vi "Write actor.vi"(8 "error in (no error)":errorcluster, 10 "actor":refnum<class "Actor.lvclass">, 11 "[MV] Key Certify in":refnum<class "[MV] Key Certify.lvclass">) -> (0 "error out":errorcluster, 3 "[MV] Key Certify out":refnum<class "[MV] Key Certify.lvclass">)   [LabVIEW 2023, in "[MV] Key Certify.lvlib" / "[MV] Key Certify.lvclass"]
uses:
  [MV] Key Certify.lvclass
  [MV] Key Certify.lvclass/[MV] Key Certify.ctl
  <vilib>/ActorFramework/Actor/Actor.lvclass
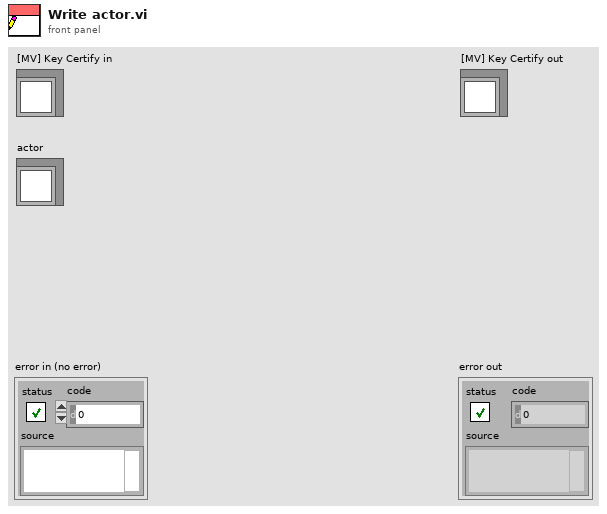
[diagram p1: front panel]
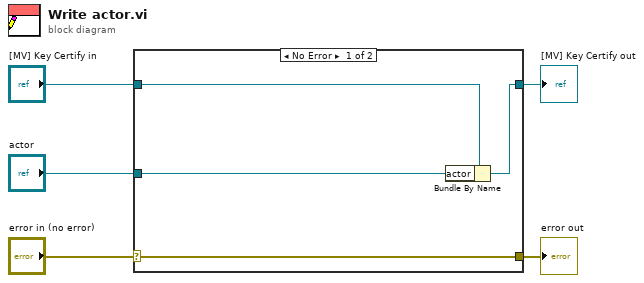
[diagram p0: block diagram]
diagram:
  n1 = case shown="No Error" "error in (no error)" {
    selector: "error in (no error)" -> [w9 w10]
    tunnel: [w9 w10] -> w4
    tunnel: [w7 w11] -> w2
    tunnel: "[MV] Key Certify in" -> [w8 w11]
    tunnel: "actor" -> [w6 _]
    frame No Error {
      n2 = Bundle By Name(cluster=w8, "actor"=w6) -> (w7:refnum<class "[MV] Key Certify.lvclass">)
    }
    frame Error {
    }
  }
  "error out" <- w4
  "[MV] Key Certify out" <- w2
